vi "Periodic Tasks.vi"(8 "error in":errorcluster) -> ()   [LabVIEW 2018]
doc: "This VI runs in parallel to other tasks. It can contain as many user-defined periodic loops as you need. These can carry out PID or other sorts of timed response."
uses:
  Refnums.vi
  <vilib>/Rock Robotics/Network Tables/NT Read Number.vi
  <vilib>/addons/control/pid/pid.llb/PID Control Input Filter (DBL).vi
  <vilib>/addons/control/pid/pid.llb/PID (DBL).vi
  LimeLight.vi
  <vilib>/addons/control/pid/NI_PID_pid.lvlib
panel:
  in  "Boolean":bool
  in  "Delay":dbl
  out "TX":dbl
  out "Correction":dbl
  in  "PID gains":T1={"proportional gain (Kc)"=0.01, "integral time (Ti, min)"=0.0, "derivative time (Td, min)"=0.0} {"proportional gain (Kc)" step=0.01}
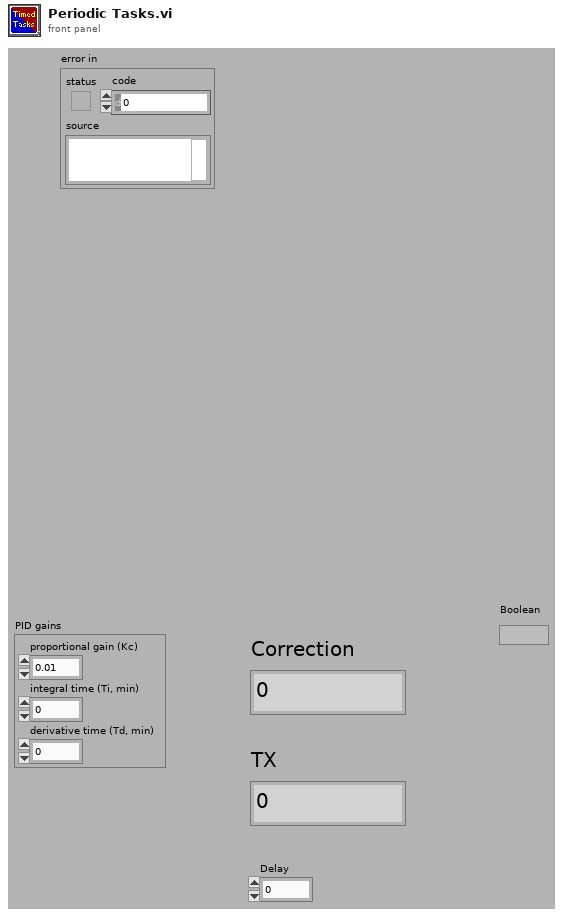
[diagram p1: front panel]
types:
  T1 = cluster{"proportional gain (Kc)":dbl, "integral time (Ti, min)":dbl, "derivative time (Td, min)":dbl}
  T2 = typedef "WPI_JoystickDevRef.ctl" = cluster{"Device":T3}
  T3 = typedef "WPI_JoystickDeviceEnum.ctl" = enum16{"USB 0", "USB 1", "USB 2", "USB 3", "USB 4", "USB 5"}
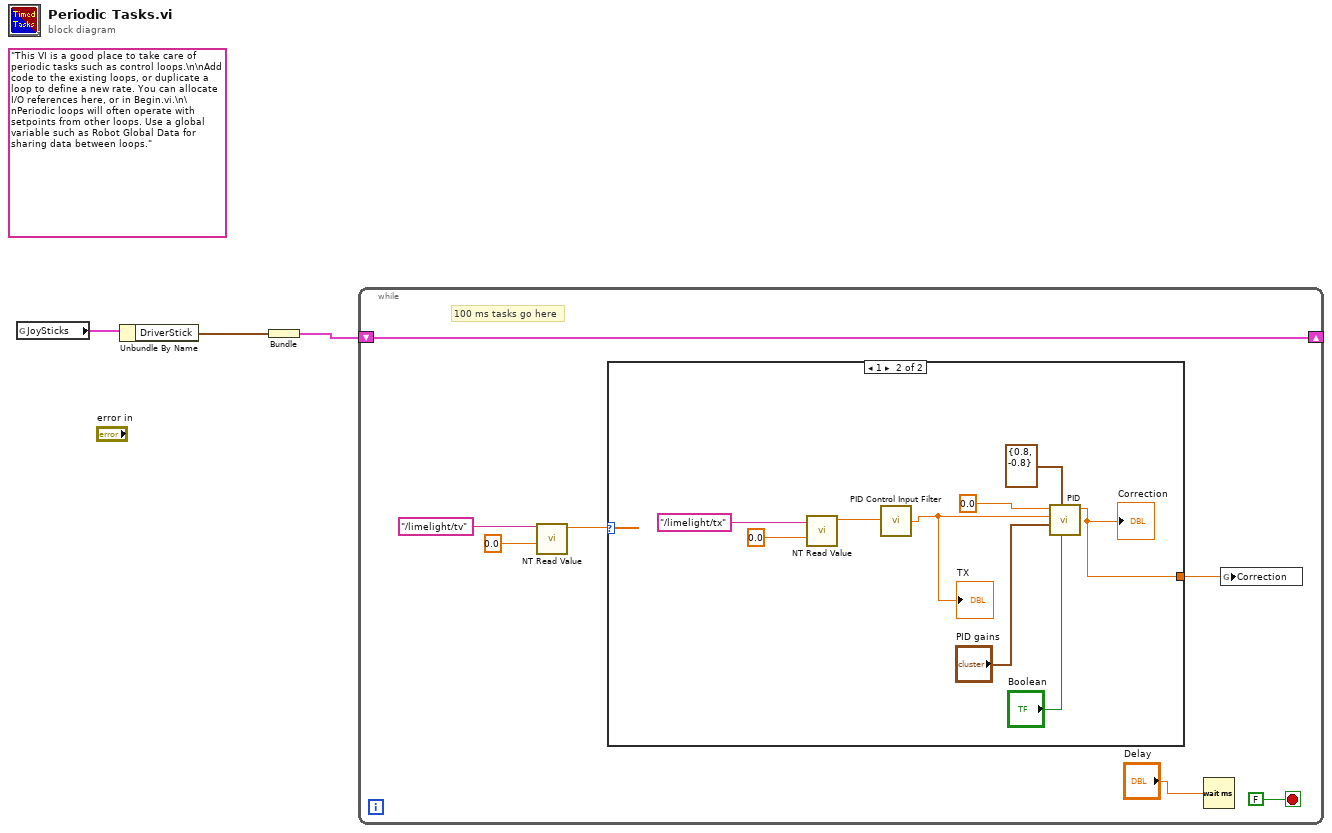
[diagram p0: block diagram]
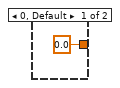
[diagram p2: hidden frame]
diagram:
  (unwired) "This VI is a good place to take care of periodic tasks such as control loops.\n\nAdd code to the existing loops, or duplicate a loop to define a new rate. You can allocate I/O references here, or in Begin.vi.\n\nPeriodic loops will often operate with setpoints from other loops. Use a global variable such as Robot Global Data for sharing data between loops."
  n1 = global read "Refnums.vi" "JoySticks"() -> (w2:cluster{"DriverStick":T2, "OperatorStick":T2})
  n2 = Unbundle By Name(w2) -> ("DriverStick"=w1:T2)
  n3 = Bundle("DriverStick"=w1) -> (w3:cluster{"DriverStick":T2})  [unwired: 1 out]
  n4 = while {
    shift-right: [w9] -> _
    shift-left: w3 -> [w9]
    stop <- FALSE stop-if-true
    # "100 ms tasks go here"
    n5 = call-poly <vilib>:"NT Read Value.vi"("Default Value"=0.0, "Name"="/limelight/tv") -> ("Numeric"=w7:dbl)  [unwired: 8 in, 1 out]
    n6 = case shown="1" w7 {
      tunnel: [0.0 ("output") w13] -> w4
      frame 0, Default {
      }
      frame 1 {
        n7 = call-poly <vilib>:"NT Read Value.vi"("Default Value"=0.0, "Name"="/limelight/tx") -> ("Numeric"=w15:dbl)  [unwired: 8 in, 1 out]
        n8 = call-poly <vilib>:"PID Control Input Filter.vi"("input"=w15) -> ("output"=w14:dbl)  [unwired: 4 in]
        "TX" <- w14
        n9 = call-poly <vilib>:"PID.vi"("reinitialize? (F)"="Boolean", "output range"=cluster{"output high":dbl, "output low":dbl} {"output high"=0.8, "output low"=-0.8}, "PID gains"="PID gains", "process variable"=w14, "setpoint"=0.0) -> ("output"=w13:dbl)  [unwired: 5 in, 1 out]
        "Correction" <- w13
      }
    }
    n10 = Wait (ms)(milliseconds to wait="Delay") -> ()  [unwired: 1 out]
    n11 = global write "LimeLight.vi" "Correction"(w4) -> ()
  }
